vi "cw_2_3.vi"() -> ()   [LabVIEW 2022 SP3]
uses:
  <vilib>/numeric/Random Number (Range) DBL.vi
panel:
  in  "stop":bool
  in  "loop delay":u32
  out "LED":bool
  in  "discrimination level":dbl step=0.1
  in  "noise amplitude":ext=0.2
  out "Waveform Chart":cluster{dbl, "discrimination level":dbl}(graph)
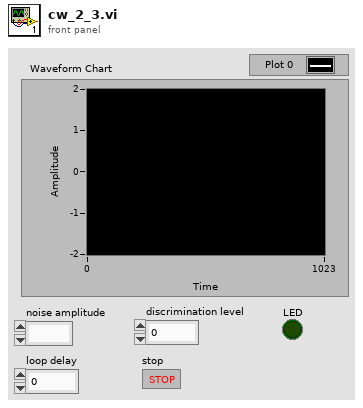
[diagram p1: front panel]
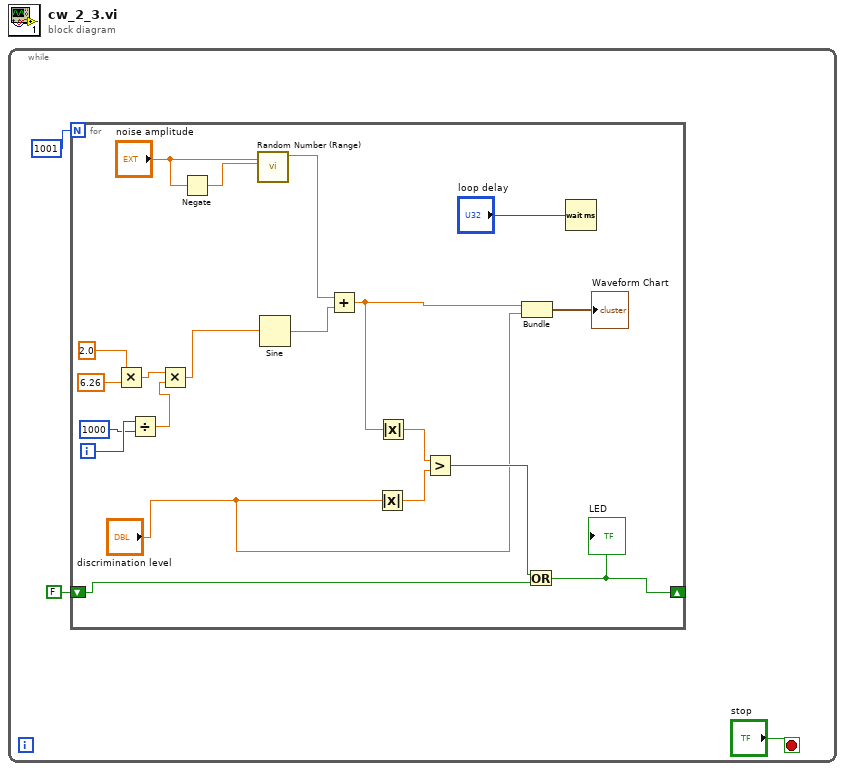
[diagram p0: block diagram]
diagram:
  n1 = while {
    stop <- "stop" stop-if-true
    n2 = for {
      N: 1001 -> [_]
      shift-right: [w7] -> _
      shift-left: FALSE -> [w9]
      i -> [w22]
      n3 = Multiply(x=2.0, y=6.26) -> (x*y=w20:dbl)
      n4 = Divide(x=w22, y=1000) -> (x/y=w19:dbl)
      n5 = Multiply(x=w20, y=w19) -> (x*y=w18:dbl)
      n6 = Negate(x="noise amplitude") -> (-x=w14:ext)
      n7 = call-poly <vilib>:"Random Number (Range).vi"("lower bound (0)"=w14, "upper bound (100)"="noise amplitude") -> ("number"=w16:dbl)  [unwired: 9 in]
      n8 = Sine(x=w18) -> (sin(x)=w17:dbl)
      n9 = Add(x=w16, y=w17) -> (x+y=w12:dbl)
      n10 = Absolute Value(x="discrimination level") -> (abs(x)=w10:dbl)
      n11 = Absolute Value(x=w12) -> (abs(x)=w11:dbl)
      n12 = Greater?(x=w11, y=w10) -> (0:w8:bool)
      n13 = Bundle(w12, "discrimination level"="discrimination level") -> (→"Waveform Chart":cluster{dbl, "discrimination level":dbl})  [unwired: 1 in]
      n14 = Or(x=w8, y=w9) -> (x .or. y?=w7:bool)
      "LED" <- w7
      n15 = Wait (ms)(milliseconds to wait="loop delay") -> ()  [unwired: 1 out]
    }
  }
